vi "displayError.vi"(8 "error in (no error)":errorcluster, 11 "ScriptEditorV2 in":refnum<class "ScriptEditorV2.lvclass">) -> (0 "error out":errorcluster, 3 "ScriptEditorV2 out":refnum<class "ScriptEditorV2.lvclass">)   [LabVIEW 2011, in "Views.lvlib" / "ScriptEditor.lvlib" / "ScriptEditorV2.lvclass"]
uses:
  ScriptEditorV2.lvclass
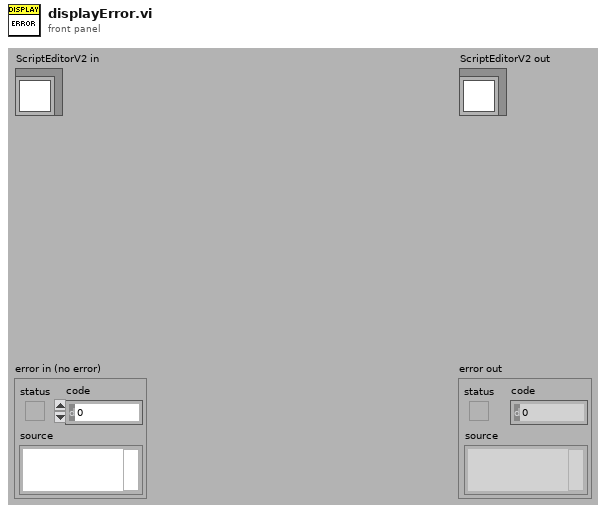
[diagram p1: front panel]
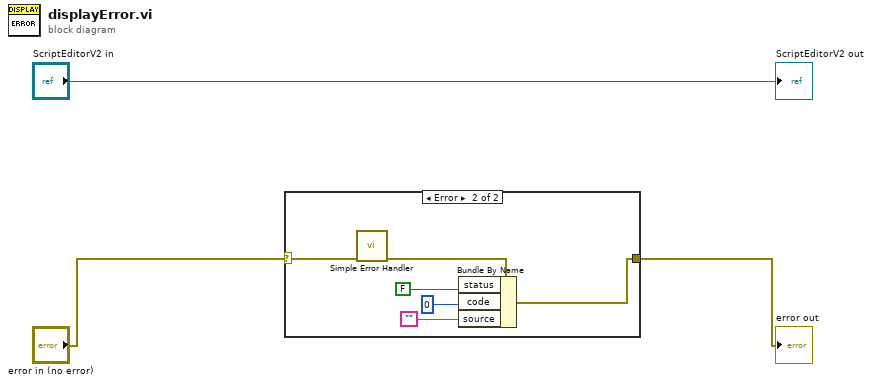
[diagram p0: block diagram]
diagram:
  n1 = case shown="Error" "error in (no error)" {
    selector: "error in (no error)" -> [w4 w10]
    tunnel: [w4 w5] -> w2
    frame No Error {
    }
    frame Error {
      n2 = call <vilib>:"Simple Error Handler.vi"("error in (no error)"=w10) -> ("error out"=w9:errorcluster)  [unwired: 4 in, 4 out]
      n3 = Bundle By Name(cluster=w9, "status"=FALSE, "code"=0, "source"="") -> (w5:errorcluster)
    }
  }
  "error out" <- w2
  "ScriptEditorV2 out" <- "ScriptEditorV2 in"
